vi "sv_Check Amplitude.vi"(11 "error in (no error)":errorcluster, 12 "amplitude":dbl format="%.2f") -> (14 "dup amplitude":dbl format="%.2f", 15 "error out":errorcluster)   [LabVIEW 2017, in "SoundVib_Distortion.lvlib"]
uses:
  <vilib>/addons/Sound and Vibration/svt_Distortion/SoundVib_Distortion.lvlib
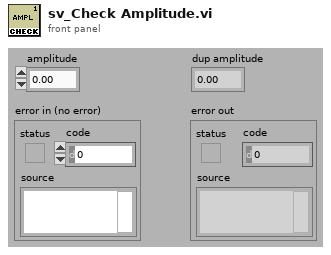
[diagram p1: front panel]
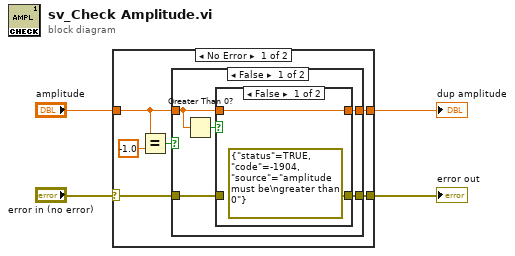
[diagram p0: block diagram]
diagram:
  n1 = case shown="No Error" "error in (no error)" {
    selector: "error in (no error)" -> [w9 w23]
    tunnel: "amplitude" -> [w7 w22]
    tunnel: [w10 w23] -> w2
    tunnel: [w5 w22] -> w4
    frame No Error {
      n2 = Equal?(x=w7, y=-1.0) -> (x = y?=w8:bool)
      n3 = case shown="False" w8 {
        tunnel: w7 -> [w11 w20]
        tunnel: w9 -> [w14 w21]
        tunnel: [w13 w21] -> w10
        tunnel: [w12 w20] -> w5
        frame False {
          n4 = Greater Than 0?(x=w11) -> (x > 0?=w15:bool)
          n5 = case shown="False" w15 {
            tunnel: [errorcluster {"status"=TRUE, "code"=-1904, "source"="amplitude must be\ngreater than 0"} ("error IO") w19] -> w13
            tunnel: w14 -> [_ w19]
            tunnel: w11 -> [w16 w18]
            tunnel: [w16 w18] -> w12
            frame False {
            }
            frame True {
            }
          }
        }
        frame True {
        }
      }
    }
    frame Error {
    }
  }
  "dup amplitude" <- w4
  "error out" <- w2
